vi "ytmsgbox.vi"(0 "Socket(From1)":i32, 1 "StopFlagRef":refnum<notifier>, 2 "JPEGPNGBMP file":path=path "C:/Users/Administrator/Desktop/无标题.png", 5 "String":string, 7 "聚焦":enum16{"无", "Btn1", "Btn2", "Btn3"}(ring), 9 "消息存在时间（s）":dbl, 11 "不可关闭":bool, 12 "按钮1文本":string, 13 "Title":string, 14 "按钮2文本":string, 15 "按钮3文本":string) -> (4 "BtnSelectOut":string)   [LabVIEW 2017]
doc: "#yyll Simple Msgbox"
uses:
  <vilib>/Utility/miscctls.llb/LVPointTypeDef.ctl
  <vilib>/Utility/miscctls.llb/LVRectTypeDef.ctl
panel:
  in  "btn1":bool
  in  "btn2":bool
  in  "btn3":bool
  out "进度条":dbl(slide)=1.0 scale=0.0..1.0
  out "String show":bool
  out "new picture":picture
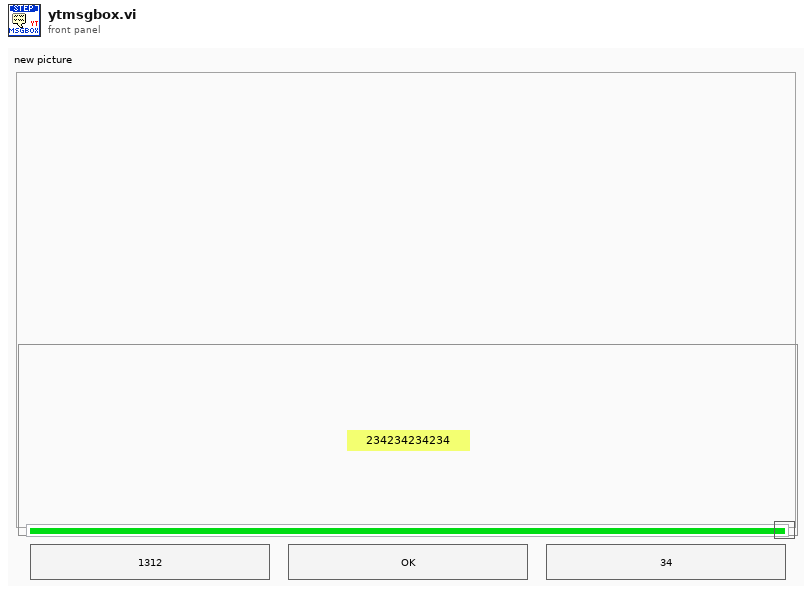
[diagram p1: front panel]
types:
  T1 = typedef "LVPointTypeDef.ctl" = cluster{"Horizontal":i16, "Vertical":i16}
  T2 = typedef "imagedata.ctl" = cluster{"image type":i32, "image depth":i32, "image":u8[], "mask":u8[], "colors":u32[], "Rectangle":cluster{"left":i16, "top":i16, "right":i16, "bottom":i16}}
  T3 = typedef "LVRectTypeDef.ctl" = cluster{"Left":i16, "Top":i16, "Right":i16, "Bottom":i16}
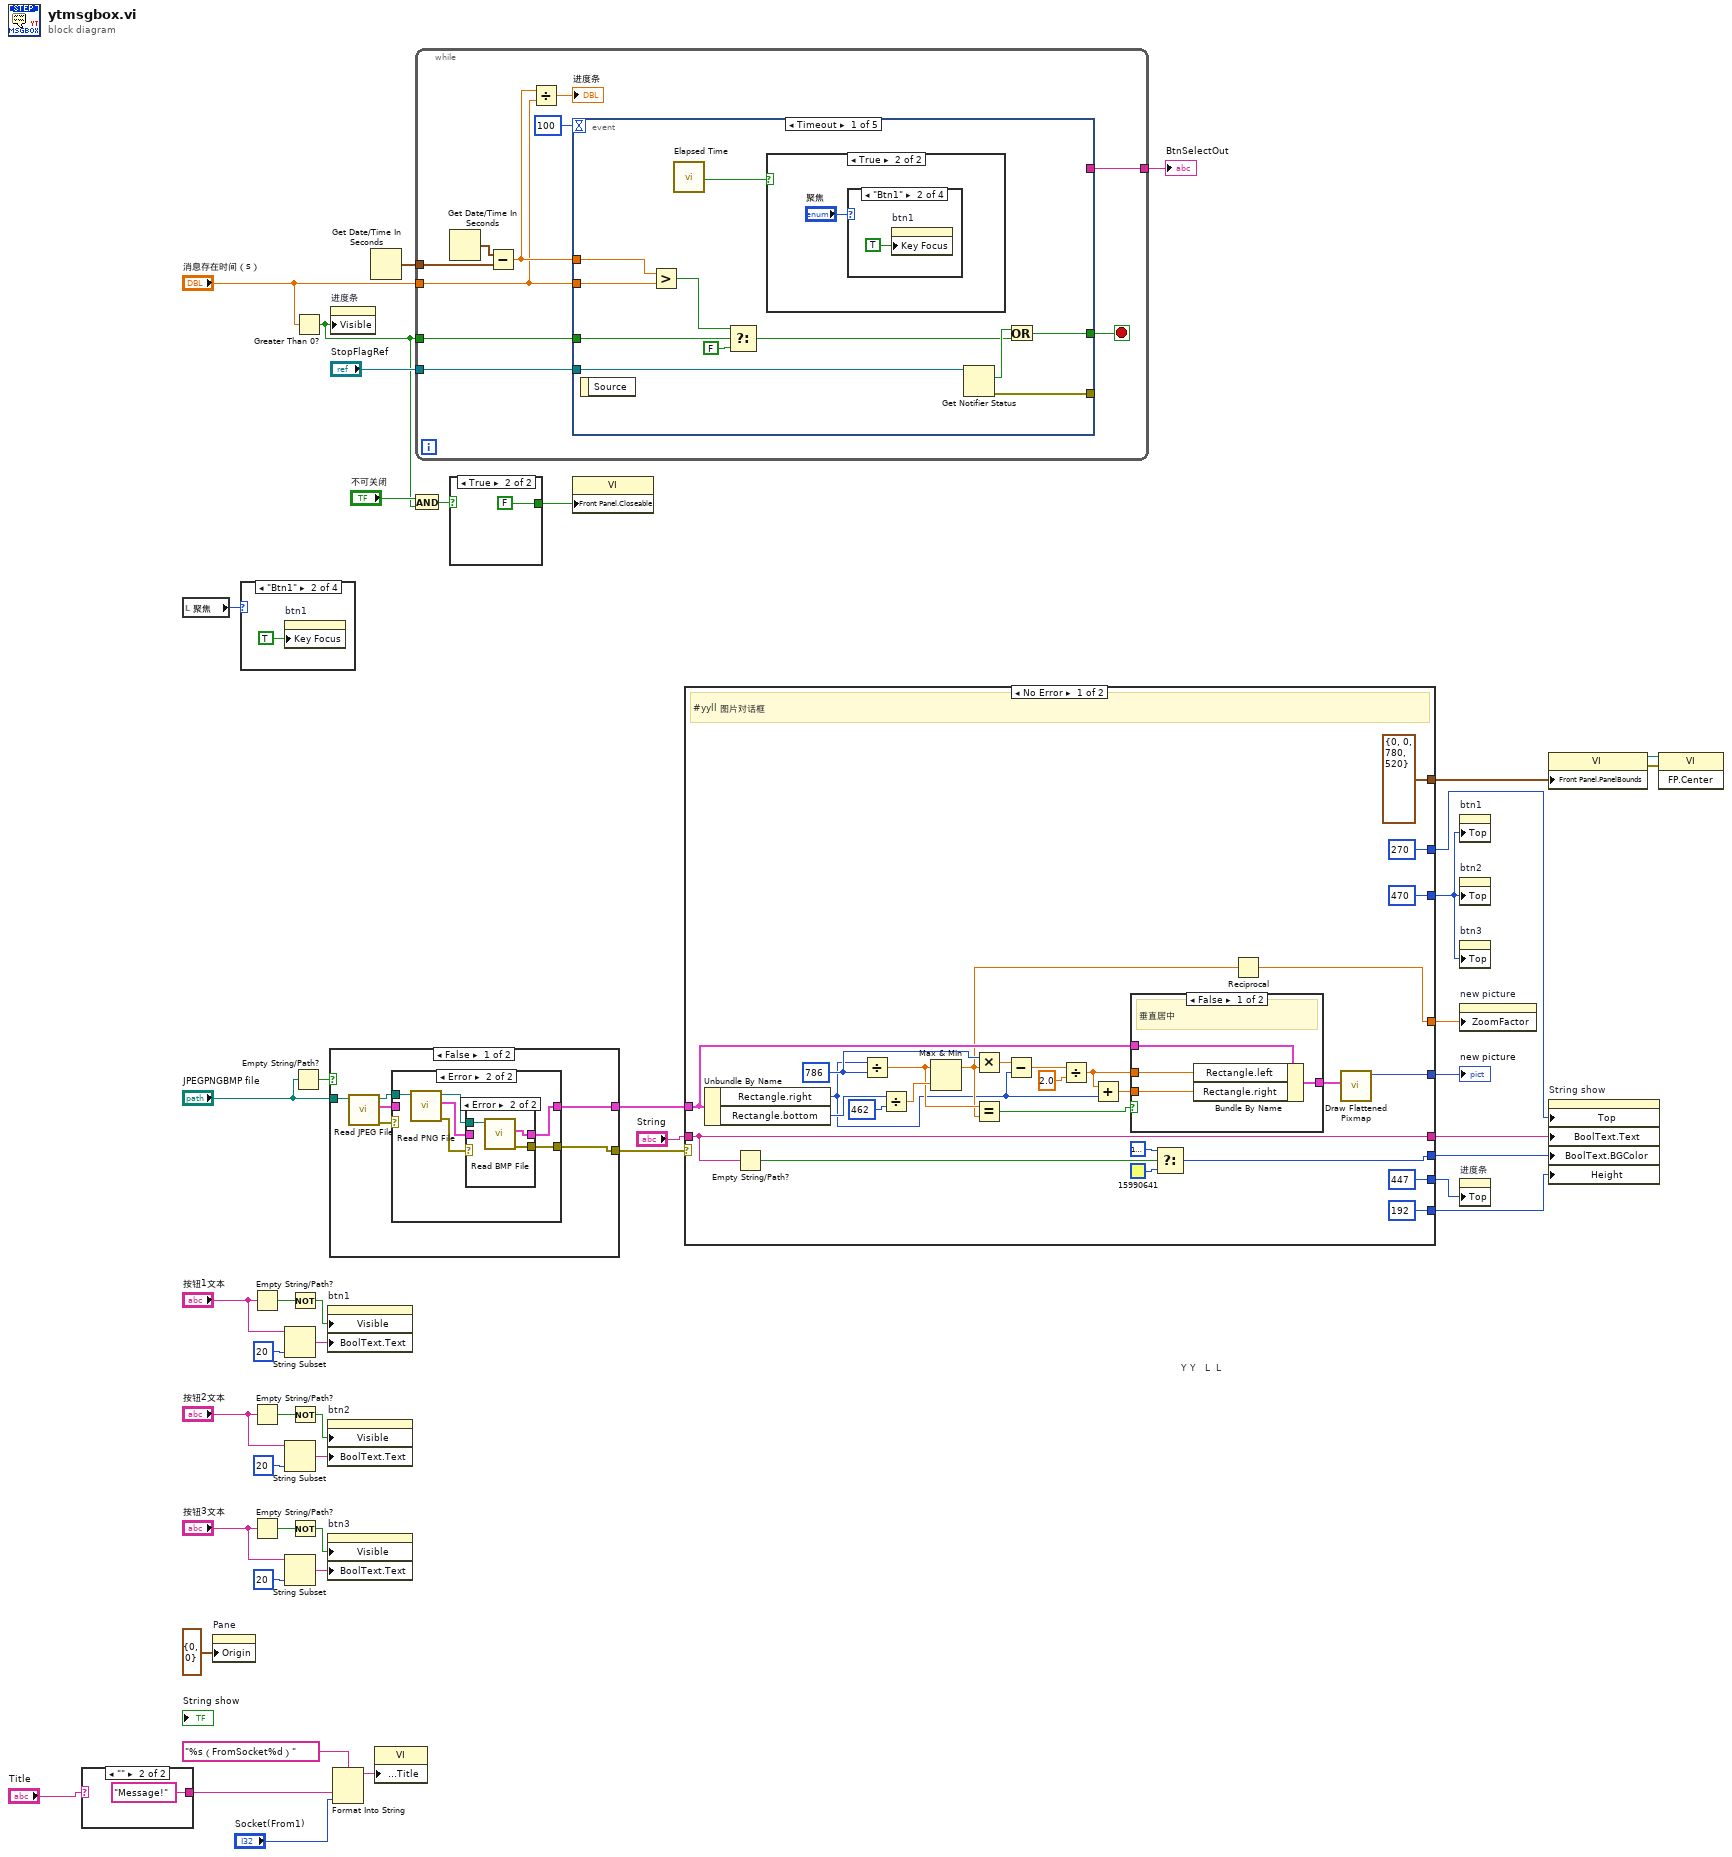
[diagram p0: block diagram]
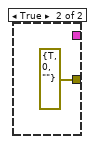
[diagram p5: hidden frame]
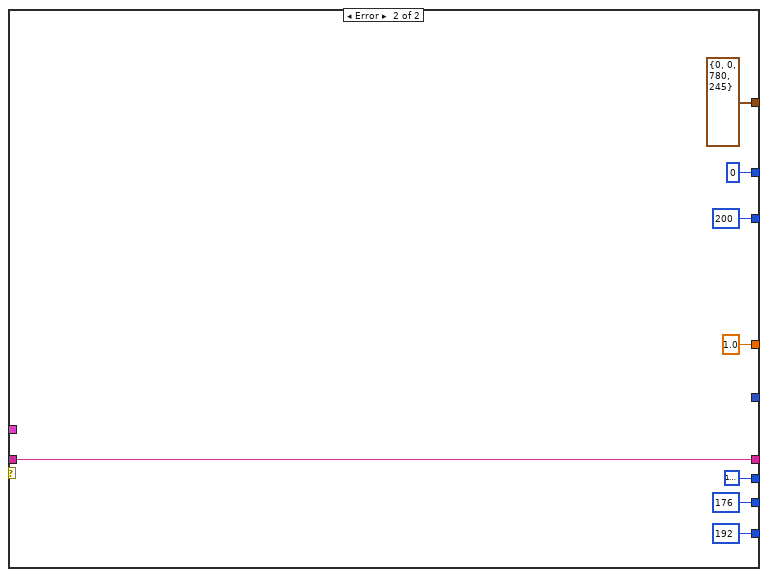
[diagram p7: hidden frame]
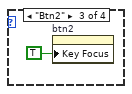
[diagram p9: hidden frame]
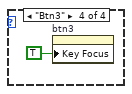
[diagram p10: hidden frame]
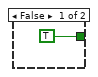
[diagram p11: hidden frame]
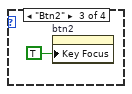
[diagram p14: hidden frame]
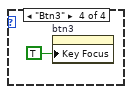
[diagram p15: hidden frame]
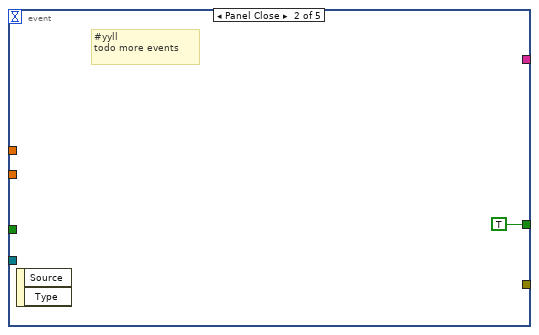
[diagram p16: hidden frame]
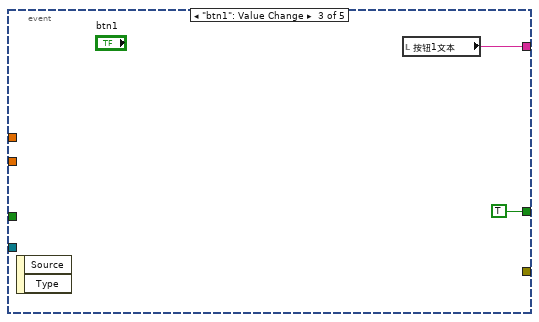
[diagram p17: hidden frame]
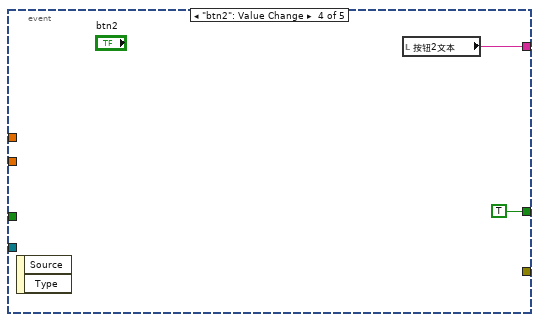
[diagram p18: hidden frame]
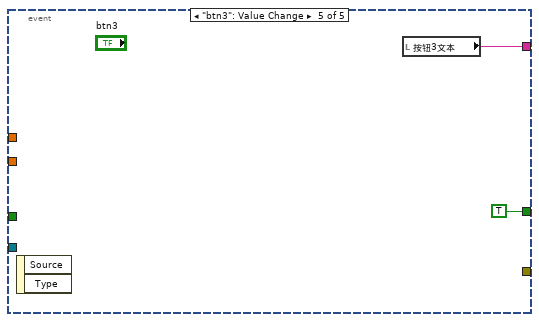
[diagram p19: hidden frame]
diagram:
  # "Y Y   L  L"
  n1 = case shown="\"\"" "Title" {
    selector: "Title" -> [w47 _]
    tunnel: [w47 "Message!"] -> w1
    frame Default {
    }
    frame "" {
    }
  }
  n2 = local read "聚焦"() -> (w21:enum16{"无", "Btn1", "Btn2", "Btn3"})
  n3 = property on="Pane" class="Pane"("Origin"=T1 {"Horizontal"=0, "Vertical"=0}) -> ()  [unwired: 2 in, 2 out]
  n4 = case shown="\"Btn1\"" w21 {
    frame "无", Default {
    }
    frame "Btn1" {
      n5 = property on="btn1" class="Bool"("Key Focus"=TRUE) -> ()  [unwired: 2 in, 2 out]
    }
    frame "Btn2" {
      n6 = property on="btn2" class="Bool"("Key Focus"=TRUE) -> ()  [unwired: 2 in, 2 out]
    }
    frame "Btn3" {
      n7 = property on="btn3" class="Bool"("Key Focus"=TRUE) -> ()  [unwired: 2 in, 2 out]
    }
  }
  n8 = Empty String/Path?(string/path="按钮1文本") -> (empty?=w36:bool)
  n9 = Empty String/Path?(string/path="按钮2文本") -> (empty?=w34:bool)
  n10 = Empty String/Path?(string/path="按钮3文本") -> (empty?=w33:bool)
  n11 = String Subset(string="按钮1文本", length (rest)=20 ("length (rest)")) -> (substring=w28:string)  [unwired: 1 in]
  n12 = String Subset(string="按钮2文本", length (rest)=20 ("length (rest)")) -> (substring=w22:string)  [unwired: 1 in]
  n13 = String Subset(string="按钮3文本", length (rest)=20 ("length (rest)")) -> (substring=w24:string)  [unwired: 1 in]
  n14 = Not(x=w36) -> (.not. x?=w35:bool)
  n15 = Not(x=w34) -> (.not. x?=w32:bool)
  n16 = Not(x=w33) -> (.not. x?=w31:bool)
  n17 = Empty String/Path?(string/path="JPEGPNGBMP file") -> (empty?=w11:bool)
  n18 = Greater Than 0?(x="消息存在时间（s）") -> (x > 0?=w37:bool)
  n19 = property on="btn1" class="Bool"("Visible"=w35, "BoolText.Text"=w28) -> ()  [unwired: 2 in, 2 out]
  n20 = property on="btn2" class="Bool"("Visible"=w32, "BoolText.Text"=w22) -> ()  [unwired: 2 in, 2 out]
  n21 = property on="btn3" class="Bool"("Visible"=w31, "BoolText.Text"=w24) -> ()  [unwired: 2 in, 2 out]
  n22 = case shown="False" w11 {
    tunnel: [w54 errorcluster {"status"=TRUE, "code"=0, "source"=""} ("error out")] -> w18
    tunnel: [w53 _] -> w17
    tunnel: "JPEGPNGBMP file" -> [w52 _]
    frame False {
      n23 = call <vilib>:"Read JPEG File.vi"("path to JPEG file"=w52) -> ("error out"=w56:errorcluster, "image data"=w57:T2, "path"=w55:path)  [unwired: 8 in]
      n24 = case shown="Error" w56 {
        tunnel: w57 -> [w58 _]
        tunnel: w55 -> [_ w64]
        tunnel: [w58 w62] -> w53
        tunnel: [_ w59] -> w54
        frame No Error {
        }
        frame Error {
          n25 = call <vilib>:"Read PNG File.vi"("path to PNG file"=w64) -> ("error out"=w63:errorcluster, "image data"=w61:T2, "path"=w60:path)  [unwired: 8 in]
          n26 = case shown="Error" w63 {
            tunnel: [w65 w67] -> w62
            tunnel: w61 -> [w65 _]
            tunnel: w60 -> [_ w68]
            tunnel: [_ w66] -> w59
            frame No Error {
            }
            frame Error {
              n27 = call <vilib>:"Read BMP File.vi"("path to BMP file"=w68) -> ("error out"=w66:errorcluster, "image data"=w67:T2)  [unwired: 8 in, 1 out]
            }
          }
        }
      }
    }
    frame True {
    }
  }
  n28 = property on="进度条" class="Slide (strict)"("Visible"=w37) -> ()  [unwired: 2 in, 2 out]
  n29 = Format Into String(format string="%s（FromSocket%d）", w1, "Socket(From1)") -> (resulting string=w46:string)  [unwired: 2 in, 1 out]
  n30 = Get Date/Time In Seconds() -> (seconds since 1Jan1904=w39:timestamp)
  n31 = property class="VI"("Front Panel.Title"=w46) -> ()  [unwired: 2 in, 2 out]
  n32 = And(x="不可关闭", y=w37) -> (x .and. y?=w42:bool)
  n33 = while {
    tunnel: "消息存在时间（s）" -> [w74]
    tunnel: w39 -> [w76]
    tunnel: "StopFlagRef" -> [w72]
    tunnel: w37 -> [w71]
    tunnel: [w70] -> w20
    stop <- w78 stop-if-true
    n34 = Get Date/Time In Seconds() -> (seconds since 1Jan1904=w77:timestamp)
    n35 = Subtract(x=w77, y=w76) -> (x-y=w75:dbl)
    n36 = Divide(x=w75, y=w74) -> (x/y=→"进度条":dbl)
    n37 = event shown="[0] Timeout" {
      selector: _ -> [_ _ _ _ _]
      dyn-events: _ -> [_ _ _ _ _]
      timeout: 100 -> [_ _ _ _ _]
      tunnel: [w86 TRUE ("Discard?") TRUE ("Discard?") TRUE ("Discard?") TRUE ("Discard?")] -> w78
      tunnel: w74 -> [w89 _ _ _ _]
      tunnel: w75 -> [w90 _ _ _ _]
      tunnel: w72 -> [w88 _ _ _ _]
      tunnel: w71 -> [w85 _ _ _ _]
      tunnel: [w80 _ _ _ _] -> _
      tunnel: [_ _ w96 w98 w100] -> w70
      event Timeout {
        n38 = event-data() -> ()  [unwired: 1 in, 1 out]
        n39 = Greater?(x=w90, y=w89) -> (0:w84:bool)
        n40 = call "Elapsed Time"() -> ("Time has Elapsed"=w81:bool)  [unwired: 12 in, 7 out]
        n41 = Select(t=w84, s=w85, f=FALSE) -> (s? t:f=w83:bool)
        n42 = case shown="True" w81 {
          frame False {
          }
          frame True {
            n43 = case shown="\"Btn1\"" "聚焦" {
              frame "无", Default {
              }
              frame "Btn1" {
                n44 = property on="btn1" class="Bool"("Key Focus"=TRUE) -> ()  [unwired: 2 in, 2 out]
              }
              frame "Btn2" {
                n45 = property on="btn2" class="Bool"("Key Focus"=TRUE) -> ()  [unwired: 2 in, 2 out]
              }
              frame "Btn3" {
                n46 = property on="btn3" class="Bool"("Key Focus"=TRUE) -> ()  [unwired: 2 in, 2 out]
              }
            }
          }
        }
        n47 = Get Notifier Status(notifier=w88) -> (current notification=w87:bool, error out=w80:errorcluster)  [unwired: 1 in, 3 out]
        n48 = Or(x=w87, y=w83) -> (x .or. y?=w86:bool)
      }
      event Panel Close {
        # "#yyll\ntodo more events"
        n49 = event-data() -> ()  [unwired: 1 in, 2 out]
      }
      event "btn1": Value Change {
        n50 = event-data() -> ()  [unwired: 1 in, 2 out]
        n51 = local read "按钮1文本"() -> (w96:string)
      }
      event "btn2": Value Change {
        n52 = event-data() -> ()  [unwired: 1 in, 2 out]
        n53 = local read "按钮2文本"() -> (w98:string)
      }
      event "btn3": Value Change {
        n54 = event-data() -> ()  [unwired: 1 in, 2 out]
        n55 = local read "按钮3文本"() -> (w100:string)
      }
    }
  }
  "BtnSelectOut" <- w20
  n56 = case shown="True" w42 {
    tunnel: [TRUE FALSE ("Front Panel Window:Closeable")] -> w41
    frame False {
    }
    frame True {
    }
  }
  n57 = property class="VI"("Front Panel.Closeable"=w41) -> ()  [unwired: 2 in, 2 out]
  n58 = case shown="No Error" w18 {
    tunnel: w17 -> [w117 _]
    tunnel: [w130 _] -> w16
    tunnel: [T3 {"Left"=0, "Top"=0, "Right"=780, "Bottom"=520} ("Front Panel Window:Panel Bounds") T3 {"Left"=0, "Top"=0, "Right"=780, "Bottom"=245} ("Front Panel Window:Panel Bounds")] -> w13
    tunnel: [i16 470 ("Bottom") i16 200 ("Bottom")] -> w10
    tunnel: [i16 192 ("Bottom") i16 192 ("Bottom")] -> w5
    tunnel: [i16 270 ("Bottom") i16 0 ("Bottom")] -> w9
    tunnel: [w122 u32 16777216] -> w8
    tunnel: [w125 w138] -> w7
    tunnel: "String" -> [w125 w138]
    tunnel: [w113 1.0] -> w4
    tunnel: [i16 447 ("Bottom") i16 176 ("Bottom")] -> w3
    frame No Error {
      w112 = i16 786 ("y")
      # "#yyll 图片对话框"
      n59 = Unbundle By Name(w117) -> ("Rectangle.right"=w106:i16, "Rectangle.bottom"=w119:i16)
      n60 = Empty String/Path?(string/path=w125) -> (empty?=w124:bool)
      n61 = Divide(x=w106, y=w112) -> (x/y=w115:dbl)
      n62 = Divide(x=w119, y=i16 462) -> (x/y=w118:dbl)
      n63 = Max & Min(x=w115, y=w118) -> (max(x,y)=w111:dbl)  [unwired: 1 out]
      n64 = Multiply(x=w112, y=w111) -> (x*y=w110:dbl)
      n65 = Equal?(x=w115, y=w111) -> (x = y?=w114:bool)
      n66 = Subtract(x=w110, y=w106) -> (x-y=w109:dbl)
      n67 = Divide(x=w109, y=2.0) -> (x/y=w107:dbl)
      n68 = Add(x=w107, y=w106) -> (x+y=w105:dbl)
      n69 = case shown="False" w114 {
        tunnel: w117 -> [w134 w135]
        tunnel: [w133 w135] -> w116
        tunnel: w107 -> [w132 _]
        tunnel: w105 -> [w131 _]
        frame False {
          # "垂直居中"
          n70 = Bundle By Name(cluster=w134, "Rectangle.left"=w132, "Rectangle.right"=w131) -> (w133:T2)
        }
        frame True {
          # "水平居中，#yyll暂不处理"
        }
      }
      n71 = Select(t=u32 16777216, s=w124, f=u32 15990641) -> (s? t:f=w122:u32)
      n72 = Reciprocal(x=w111) -> (1/x=w113:dbl)
      n73 = call <vilib>:"Draw Flattened Pixmap.vi"("image data"=w116) -> ("new picture"=w130:picture)  [unwired: 8 in]
    }
    frame Error {
    }
  }
  "new picture" <- w16
  n74 = property on="btn1" class="Bool"("Top"=w10) -> ()  [unwired: 2 in, 2 out]
  n75 = property on="btn2" class="Bool"("Top"=w10) -> ()  [unwired: 2 in, 2 out]
  n76 = property on="btn3" class="Bool"("Top"=w10) -> ()  [unwired: 2 in, 2 out]
  n77 = property on="new picture" class="Pict"("ZoomFactor"=w4) -> ()  [unwired: 2 in, 2 out]
  n78 = property on="进度条" class="Slide (strict)"("Top"=w3) -> ()  [unwired: 2 in, 2 out]
  n79 = property class="VI"("Front Panel.PanelBounds"=w13) -> (reference out=w15:refnum<vi>, error out=w14:errorcluster)  [unwired: 2 in]
  n80 = property on="String show" class="Bool"("Top"=w9, "BoolText.Text"=w7, "BoolText.BGColor"=w8, "Height"=w5) -> ()  [unwired: 2 in, 2 out]
  n81 = invoke class="VI" method="FP.Center"(reference=w15, error in=w14) -> ()  [unwired: 1 in, 3 out]
